vi "set_exponential_intensity.vi"(8 "error in (no error)":errorcluster, 10 "power slider in":cluster{dbl, dbl}, 11 "number of frames":i32) -> (0 "error out":errorcluster, 3 "amplitude out":u16[](array[numeric]))   [LabVIEW 2010, in "TrajectoryMH100122AODRAPS.lvclass"]
uses:
  TrajectoryMH100122AODRAPS.lvclass
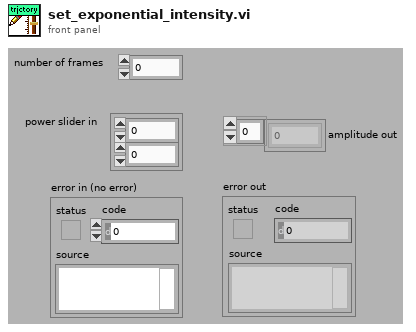
[diagram p1: front panel]
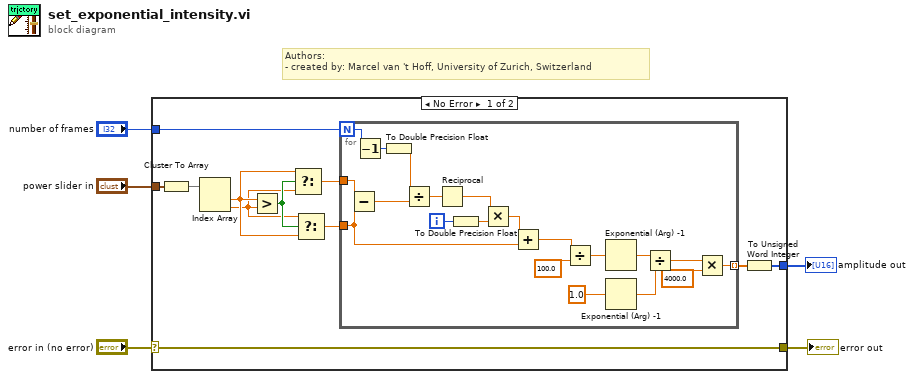
[diagram p0: block diagram]
diagram:
  # "Authors: \n- created by: Marcel van 't Hoff, University of Zurich, Switzerland"
  n1 = case shown="No Error" "error in (no error)" {
    selector: "error in (no error)" -> [w7 w37]
    tunnel: [w16 _] -> w5
    tunnel: "number of frames" -> [w10 _]
    tunnel: "power slider in" -> [w8 _]
    tunnel: [w7 w37] -> w1
    frame No Error {
      n2 = Cluster To Array(cluster=w8) -> (array=w9:dbl[])
      n3 = Index Array(array=w9) -> (element #1=w12:dbl, element #2=w11:dbl)  [unwired: 2 in]
      n4 = Greater?(x=w12, y=w11) -> (0:w13:bool)
      n5 = Select(t=w12, s=w13, f=w11) -> (s? t:f=w14:dbl)
      n6 = Select(t=w11, s=w13, f=w12) -> (s? t:f=w15:dbl)
      n7 = for {
        N: w10 -> [w30]
        tunnel: w14 -> [w34]
        tunnel: w15 -> [w18]
        tunnel: [w31] -> w6 mode=indexing
        i -> [w33]
        n8 = Subtract(x=w34, y=w18) -> (x-y=w28:dbl)
        n9 = Decrement(x=w30) -> (x-1=w29:i32)
        n10 = To Double Precision Float(number=w29) -> (double precision float=w27:dbl)
        n11 = Divide(x=w27, y=w28) -> (x/y=w26:dbl)
        n12 = Reciprocal(x=w26) -> (1/x=w25:dbl)
        n13 = To Double Precision Float(number=w33) -> (double precision float=w24:dbl)
        n14 = Multiply(x=w25, y=w24) -> (x*y=w19:dbl)
        n15 = Add(x=w19, y=w18) -> (x+y=w17:dbl)
        n16 = Divide(x=w17, y=100.0) -> (x/y=w35:dbl)
        n17 = Exponential (Arg) -1(1:w35) -> (0:w22:dbl)
        n18 = Exponential (Arg) -1(1:1.0 ("y")) -> (0:w21:dbl)
        n19 = Divide(x=w22, y=w21) -> (x/y=w20:dbl)
        n20 = Multiply(x=w20, y=4000.0) -> (x*y=w31:dbl)
      }
      n21 = To Unsigned Word Integer(number=w6) -> (unsigned 16bit integer=w16:u16[])
    }
    frame Error {
    }
  }
  "amplitude out" <- w5
  "error out" <- w1
